vi "Read Script Name.vi"(11 "CI Project in":refnum<class "CI Project.lvclass">) -> (2 "Script Name":string)   [LabVIEW 2014, in "CI Project.lvclass"]
uses:
  CI Project.lvclass
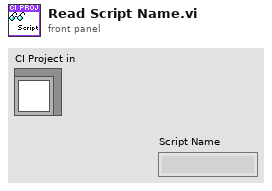
[diagram p1: front panel]
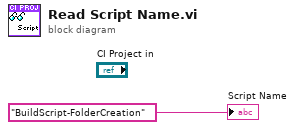
[diagram p0: block diagram]
diagram:
  "Script Name" <- "BuildScript-FolderCreation" ("Script Name")
